vi "Set 1D Array Double.vi"(5 "use temporary file? (F)":bool, 7 "column vector?":bool, 8 "error in":errorcluster, 9 "value":dbl[](array[numeric]), 10 "variable name":string, 11 "GOLPI ref. in":T1={"pipe handle"={"lv_proc.dll file path"=path "", "process instance handle"=[], "debug mode"=FALSE, "debug data"=[]}, "fast read timeout [ms]"=500, "fast read settle time [ms]"=10, "fast read to multiple [ms]"=1, "max elements per input line"=100, "slow read timeout [ms]"=5000, "stdin double format specifier"="%_16e", "max elements per stdout output column"=100, "console mode bitstream"=FALSE, "bitstream first read timeout [ms]"=1000, "bitstream read timeout [ms]"=50, "struct transfer possible"=FALSE, "matlab mode"=FALSE}) -> (0 "error out":errorcluster, 3 "GOLPI ref. out":T1={"pipe handle"={"lv_proc.dll file path"=path "", "process instance handle"=[], "debug mode"=FALSE, "debug data"=[]}, "fast read timeout [ms]"=500, "fast read settle time [ms]"=10, "fast read to multiple [ms]"=1, "max elements per input line"=100, "slow read timeout [ms]"=5000, "stdin double format specifier"="%_16e", "max elements per stdout output column"=100, "console mode bitstream"=FALSE, "bitstream first read timeout [ms]"=1000, "bitstream read timeout [ms]"=50, "struct transfer possible"=FALSE, "matlab mode"=FALSE})   [LabVIEW 2020, in "GOLPI library.lvlib"]
doc: "Part of polymorph Set Variable.vi"
uses:
  GOLPI library.lvlib
  GOLPI reference Type Def.ctl
  Pipe Handle.ctl
  LV Process library.lvlib
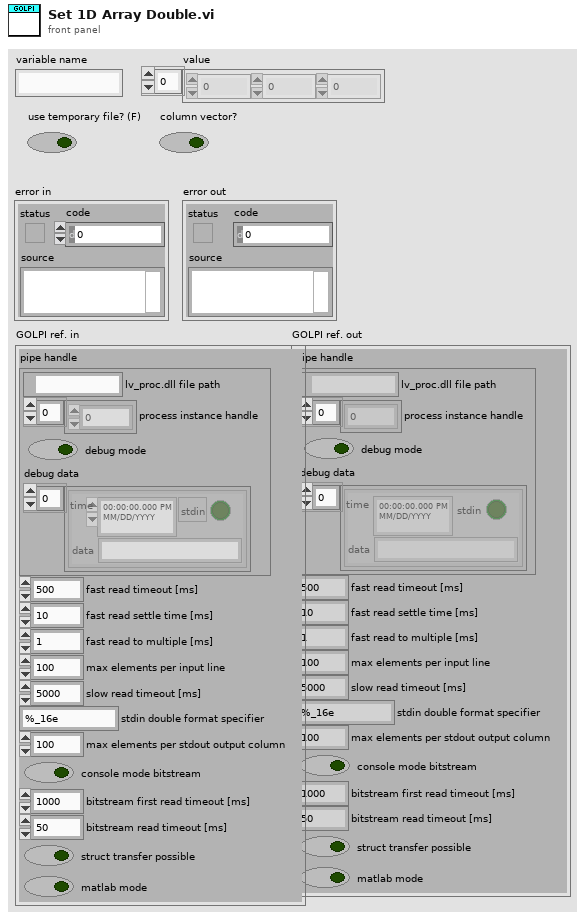
[diagram p1: front panel]
types:
  T1 = typedef "GOLPI library.lvlib/GOLPI reference Type Def.ctl" = cluster{"pipe handle":T2, "fast read timeout [ms]":u32, "fast read settle time [ms]":u32, "fast read to multiple [ms]":u32, "max elements per input line":u32, "slow read timeout [ms]":u32, "stdin double format specifier":string, "max elements per stdout output column":u32, "console mode bitstream":bool, "bitstream first read timeout [ms]":u32, "bitstream read timeout [ms]":u32, "struct transfer possible":bool, "matlab mode":bool}
  T2 = typedef "LV Process library.lvlib/Pipe Handle.ctl" = cluster{"lv_proc.dll file path":path, "process instance handle":u32[], "debug mode":bool, "debug data":cluster{"time":timestamp, "stdin":bool, "data":string}[]}
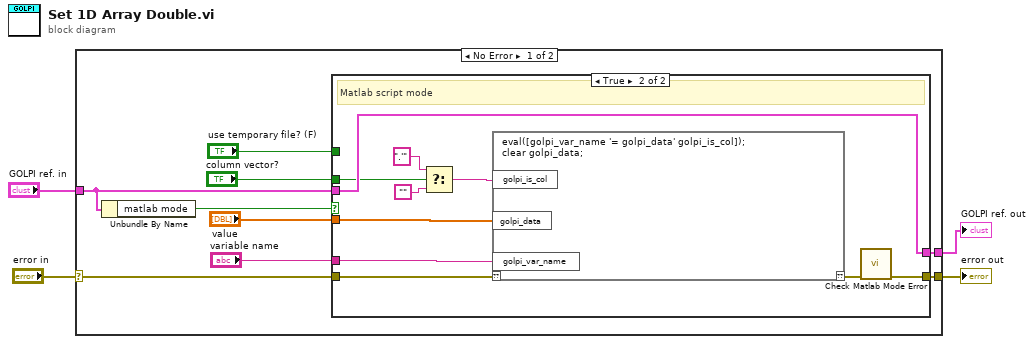
[diagram p0: block diagram]
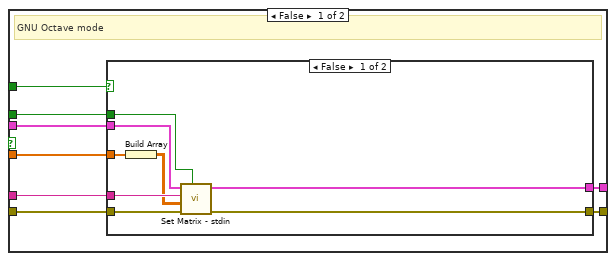
[diagram p2: hidden frame]
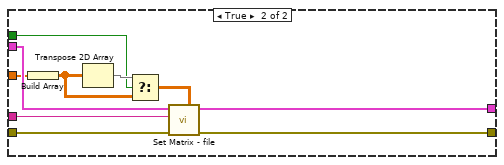
[diagram p3: hidden frame]
diagram:
  n1 = case shown="No Error" "error in" {
    selector: "error in" -> [w12 w51]
    tunnel: [w11 w51] -> w4
    tunnel: "GOLPI ref. in" -> [w6 w50]
    tunnel: [w10 w50] -> w1
    frame No Error {
      n2 = Unbundle By Name(w6) -> ("matlab mode"=w5:bool)
      n3 = case shown="True" w5 {
        tunnel: "variable name" -> [w21 w48]
        tunnel: w12 -> [w20 w49]
        tunnel: [w19 w40] -> w11
        tunnel: w6 -> [w18 w46]
        tunnel: [w17 w46] -> w10
        tunnel: "value" -> [w16 w47]
        tunnel: "column vector?" -> [w15 w45]
        tunnel: "use temporary file? (F)" -> [w14 _]
        frame False {
          # "GNU Octave mode"
          n4 = case shown="False" w14 {
            tunnel: w21 -> [w29 w39]
            tunnel: w20 -> [w28 w38]
            tunnel: [w27 w35] -> w19
            tunnel: w18 -> [w26 w37]
            tunnel: [w25 w36] -> w17
            tunnel: w16 -> [w24 w32]
            tunnel: w15 -> [w22 w31]
            frame False {
              n5 = Build Array(w24) -> (w23:dbl[][])
              n6 = call "Set Matrix - stdin.vi"("swap dimensions? (F)"=w22, "error in"=w28, "value"=w23, "variable name"=w29, "GOLPI ref. in"=w26) -> ("error out"=w27:errorcluster, "GOLPI ref. out"=w25:T1)  [unwired: 5 in]
            }
            frame True {
              n7 = Build Array(w32) -> (w34:dbl[][])
              n8 = Transpose 2D Array(2D array=w34) -> (transposed array=w33:dbl[][])
              n9 = Select(t=w33, s=w31, f=w34) -> (s? t:f=w30:dbl[][])
              n10 = call "Set Matrix - file.vi"("double array"=w30, "error in (no error)"=w38, "variable name"=w39, "GOLPI ref. in"=w37) -> ("error out"=w35:errorcluster, "GOLPI ref. out"=w36:T1)  [unwired: 6 in]
            }
          }
        }
        frame True {
          # "Matlab script mode"
          n11 = Select(t=".'", s=w45, f="") -> (s? t:f=w44:string)
          n12 = script code="eval([golpi_var_name '= golpi_data' golpi_is_col]);\nclear golpi_data;"("??"=w49, "golpi_var_name"=w48, "golpi_data"=w47, "golpi_is_col"=w44) -> ("??"=w41:errorcluster)
          n13 = call "Check Matlab Mode Error.vi"("error in"=w41) -> ("error out"=w40:errorcluster)  [unwired: 10 in]
        }
      }
    }
    frame Error {
    }
  }
  "error out" <- w4
  "GOLPI ref. out" <- w1
